vi "0xE2_Write_one_parameter_of_type_int_by_ID.vi"(8 "error in":errorcluster, 9 "ParamIn":i32, 10 "ID_IntParam":string, 11 "paramUnicorn":T1={"conParam"={"ReadIntParam"=FALSE, "ReadDescrParam"=FALSE, "ReadFloatParam"=FALSE, "debug"=FALSE, "ReadJSON"=FALSE, "IP_address"="", "N_attempts"=0, "type_con"=enum."Serial", "MB_address"=0, "VISA"="", "connection ID"=refnum, "nameDevices"="", "timeout"=0, "port"=0, "type_version"="", "baud_rate"=0, "VersionControl"=FALSE, "TCP_conn"=FALSE, "WindowSize"=700}, "Param"={"NumParam"={"NTelem"=0, "NInt"=0, "NFloat"=0, "NTable"=0}, "ParamInt"=[], "Telemetry"=[], "Table"=[], "ParamFloat"=[]}}) -> (0 "error out":errorcluster, 1 "NumParam":i32, 3 "paramUnicornOut":T1={"conParam"={"ReadIntParam"=FALSE, "ReadDescrParam"=FALSE, "ReadFloatParam"=FALSE, "debug"=FALSE, "ReadJSON"=FALSE, "IP_address"="", "N_attempts"=0, "type_con"=enum."Serial", "MB_address"=0, "VISA"="", "connection ID"=refnum, "nameDevices"="", "timeout"=0, "port"=0, "type_version"="", "baud_rate"=0, "VersionControl"=FALSE, "TCP_conn"=FALSE, "WindowSize"=700}, "Param"={"NumParam"={"NTelem"=0, "NInt"=0, "NFloat"=0, "NTable"=0}, "ParamInt"=[], "Telemetry"=[], "Table"=[], "ParamFloat"=[]}})   [LabVIEW 2017, in "LV_Unicorn.lvlib"]
uses:
  LV_Unicorn.lvlib
  Control/unicorn_Param.ctl
  Control/unicorn_conn.ctl
  Control/unicorn_JSON.ctl
  Control/unicorn_ParamInt.ctl
  Control/unicorn_Telemetry.ctl
  Control/unicorn_Table.ctl
  Control/unicorn_ParamFloat.ctl
panel:
  out "ParamOut":i32
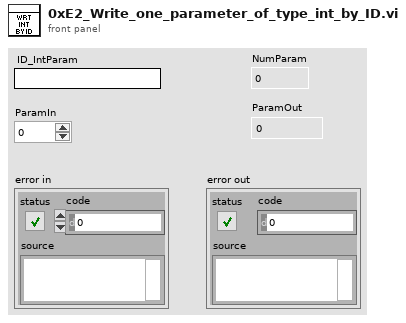
[diagram p1: front panel]
types:
  T1 = typedef "LV_Unicorn.lvlib/unicorn_Param.ctl" = cluster{"conParam":T2, "Param":T3}
  T2 = typedef "LV_Unicorn.lvlib/unicorn_conn.ctl" = cluster{"ReadIntParam":bool, "ReadDescrParam":bool, "ReadFloatParam":bool, "debug":bool, "ReadJSON":bool, "IP_address":string, "N_attempts":i32, "type_con":enum16{"Serial", "TCP"}, "MB_address":i32, "VISA":refnum<visa-resource-name>, "connection ID":refnum<k5>, "nameDevices":string, "timeout":i32, "port":u16, "type_version":string, "baud_rate":u32, "VersionControl":bool, "TCP_conn":bool, "WindowSize":i32}
  T3 = typedef "LV_Unicorn.lvlib/unicorn_JSON.ctl" = cluster{"NumParam":cluster{"NTelem":i32, "NInt":i32, "NFloat":i32, "NTable":i32}, "ParamInt":T4, "Telemetry":T5, "Table":T6, "ParamFloat":T7}
  T4 = typedef "LV_Unicorn.lvlib/unicorn_ParamInt.ctl" = cluster{"ID":string, "Num":i32, "Name":string, "Type":string, "Enum":string, "Desc":string, "Unit":string, "Access":string, "FormatStr":string, "Min":i32, "Max":i32}[]
  T5 = typedef "LV_Unicorn.lvlib/unicorn_Telemetry.ctl" = cluster{"ID":string, "Num":i32, "Name":string, "Desc":string, "Unit":string, "FormatStr":string, "Min":i32, "Max":i32}[]
  T6 = typedef "LV_Unicorn.lvlib/unicorn_Table.ctl" = cluster{"Num":i32, "Access":string, "ColumnCount":i32, "NeedParamPrepare":bool, "Columns":cluster{"Column":i32, "Desc":string, "Name":string}[], "DataType":string, "FormatStr":string, "ID":string, "Name":string, "RowCount":i32, "Rows":cluster{"Desc":string, "ID":string, "Max":i32, "Min":i32, "Name":string, "Row":i32, "Unit":string}[], "Type":string}[]
  T7 = typedef "LV_Unicorn.lvlib/unicorn_ParamFloat.ctl" = cluster{"ID":string, "Num":i32, "Name":string, "Type":string, "Enum":string, "Desc":string, "Unit":string, "Access":string, "FormatStr":string, "Min":sgl, "Max":sgl}[]
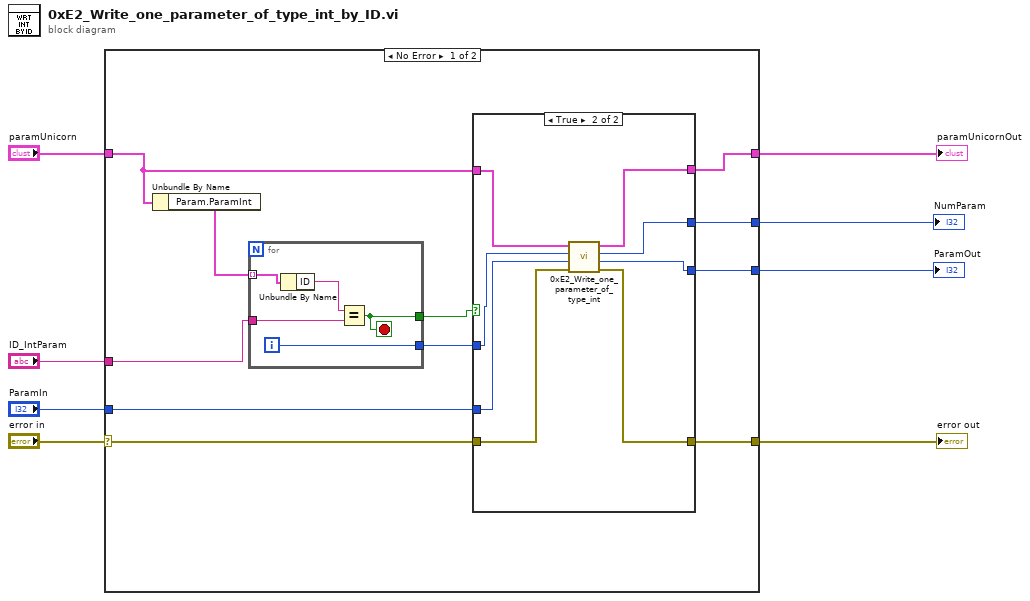
[diagram p0: block diagram]
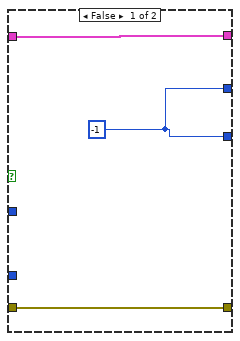
[diagram p2: hidden frame]
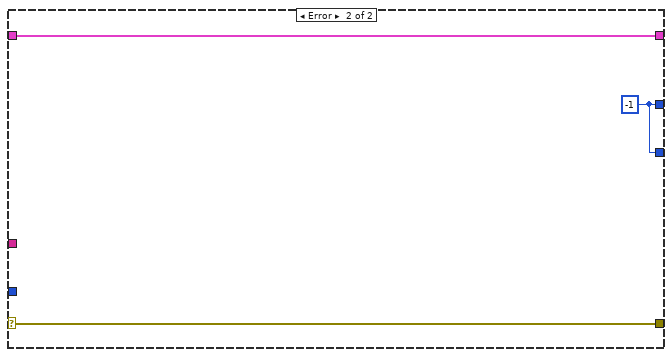
[diagram p3: hidden frame]
diagram:
  n1 = case shown="No Error" "error in" {
    selector: "error in" -> [w13 w38]
    tunnel: [w19 w37] -> w8
    tunnel: "ParamIn" -> [w18 _]
    tunnel: "paramUnicorn" -> [w17 w37]
    tunnel: [w16 w38] -> w5
    tunnel: [w15 w36] -> w4
    tunnel: [w14 w36] -> w3
    tunnel: "ID_IntParam" -> [w11 _]
    frame No Error {
      n2 = Unbundle By Name(w17) -> ("Param.ParamInt"=w12:T4)
      n3 = for {
        tunnel: w11 -> [w22]
        tunnel: [w21] -> w9
        tunnel: w12 -> [w24] mode=indexing
        tunnel: [w20] -> w10
        i -> [w21]
        stop <- w20 stop-if-true
        n4 = Unbundle By Name(w24) -> ("ID"=w23:string)
        n5 = Equal?(x=w23, y=w22) -> (x = y?=w20:bool)
      }
      n6 = case shown="True" w10 {
        tunnel: [w26 w35] -> w16
        tunnel: w17 -> [w27 w34]
        tunnel: w18 -> [_ w33]
        tunnel: [w27 w32] -> w19
        tunnel: w13 -> [w26 w31]
        tunnel: [w25 w30] -> w15
        tunnel: [w25 w29] -> w14
        tunnel: w9 -> [_ w28]
        frame False {
          w25 = -1
        }
        frame True {
          n7 = call "0xE2_Write_one_parameter_of_type_int.vi"("error in"=w31, "ParamIn"=w33, "NumParamIn"=w28, "paramUnicorn 2"=w34) -> ("error out"=w35:errorcluster, "ParamOut"=w29:i32, "NumParamOut"=w30:i32, "paramUnicornOut"=w32:T1)  [unwired: 4 in]
        }
      }
    }
    frame Error {
      w36 = -1 ("NumParamOut")
    }
  }
  "paramUnicornOut" <- w8
  "NumParam" <- w4
  "error out" <- w5
  "ParamOut" <- w3
